vi "Create VIPC from folder.vi"(8 "error in (no error)":errorcluster, 10 "Dependency folder relative path":string="tooling\\unit tests", 11 "Project path":path) -> (0 "error out":errorcluster)   [LabVIEW 2021]
uses:
  <vilib>/AppBuilder/AB_API_Simple/NI_App_Builder_API.lvlib
  <vilib>/JKI/VIPM API/VIPM API_vipm_api.lvlib
  <vilib>/AppBuilder/AB_API_Simple/Get Build Specification Version (path).vi
  <vilib>/AppBuilder/AB_API_Simple/Build (path).vi
panel:
  out "appended path":path
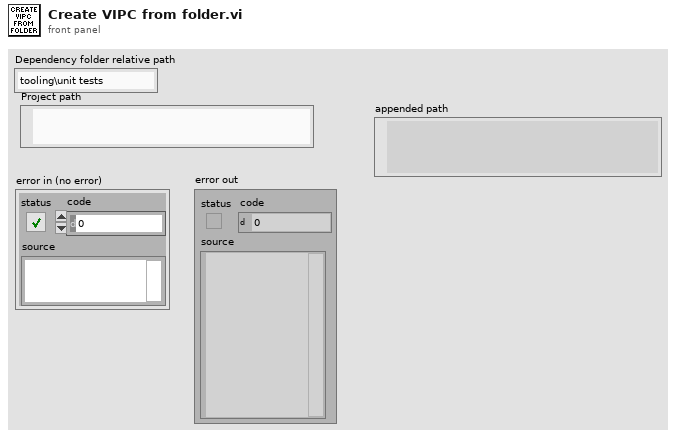
[diagram p1: front panel]
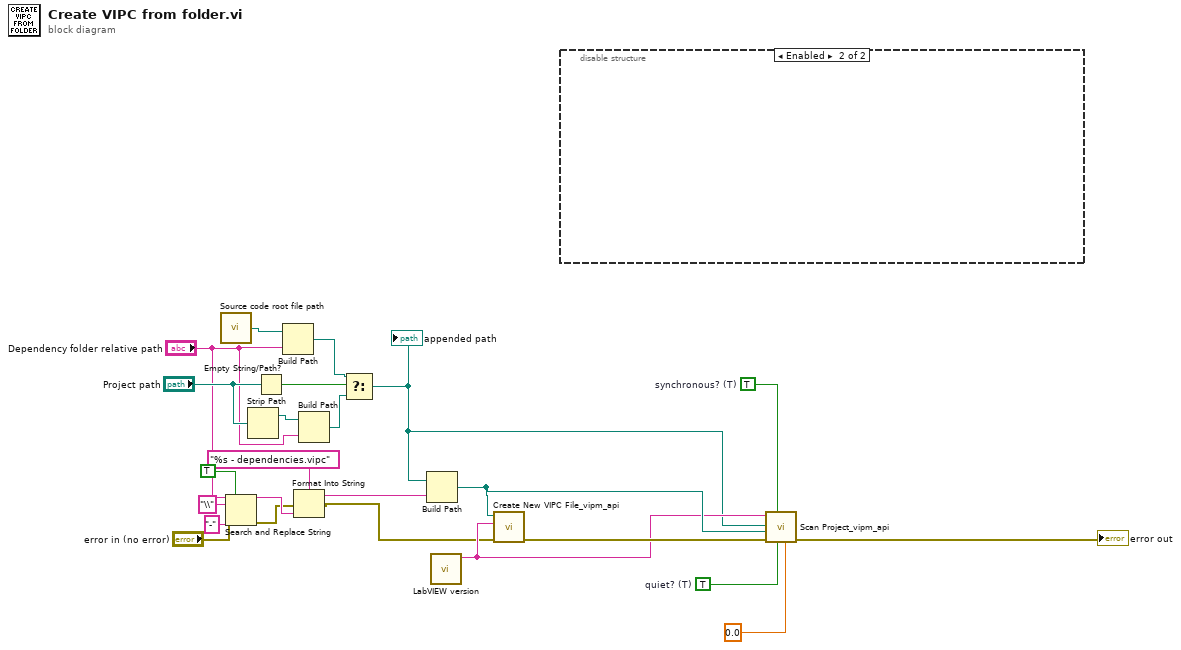
[diagram p0: block diagram]
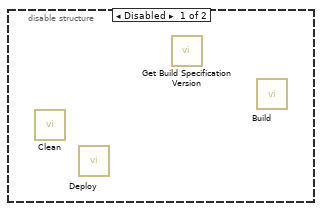
[diagram p2: hidden frame]
diagram:
  w23 = TRUE  # synchronous? (T)
  w24 = TRUE  # quiet? (T)
  n1 = call "Source code root file path.vi"() -> ("Source code root path"=w18:path)  [unwired: 1 in]
  n2 = Search and Replace String(replace all?=TRUE ("replace all? (F)"), input string="Dependency folder relative path", search string="\\", replace string="-" ("replace string (\"\")"), error in="error in (no error)") -> (result string=w11:string, error out=w6:errorcluster)  [unwired: 3 in, 2 out]
  n3 = Strip Path(path="Project path") -> (stripped path=w3:path)  [unwired: 1 out]
  n4 = Empty String/Path?(string/path="Project path") -> (empty?=w17:bool)
  n5 = Build Path(base path=w18, name or relative path="Dependency folder relative path") -> (appended path=w16:path)
  n6 = Format Into String(format string="%s - dependencies.vipc" ("LabVIEW Version"), error in=w6, w11) -> (resulting string=w12:string, error out=w5:errorcluster)  [unwired: 1 in]
  n7 = Build Path(base path=w3, name or relative path="Dependency folder relative path") -> (appended path=w2:path)
  n8 = Select(t=w16, s=w17, f=w2) -> (s? t:f=w4:path)
  "appended path" <- w4
  n9 = Build Path(base path=w4, name or relative path=w12) -> (appended path=w20:path)
  n10 = call "LabVIEW version.vi"() -> ("Application:Version Year with bitness"=w15:string)  [unwired: 11 in]
  n11 = call <vilib>:"Create New VIPC File_vipm_api.vi"("error in (no error)"=w5, "LabVIEW Version"=w15, "Path to New VIPC File"=w20) -> ("error out"=w22:errorcluster)  [unwired: 8 in]
  n12 = disable-structure shown="Enabled" {
    frame Disabled {
      n13 = call <vilib>:"Clean.vi"() -> ()  [unwired: 11 in, 1 out]
      n14 = call <vilib>:"Deploy.vi"() -> ()  [unwired: 11 in, 1 out]
      n15 = call-poly <vilib>:"Get Build Specification Version.vi"() -> ()  [unwired: 10 in, 2 out]
      n16 = call-poly <vilib>:"Build.vi"() -> ()  [unwired: 10 in, 2 out]
    }
    frame Enabled {
    }
  }
  n17 = call <vilib>:"Scan Project_vipm_api.vi"("Timeout in seconds (0: no timeout)"=0.0, "quiet? (T)"=w24, "synchronous? (T)"=w23, "error in (no error)"=w22, "Path to VIPC File"=w20, "Project file, VI or project dir path"=w4, "LabVIEW Version"=w15) -> ("error out"=→"error out":errorcluster)  [unwired: 4 in]
